vi "Format UI Size.vi"() -> (0 "error out":errorcluster)   [LabVIEW 2015, in "Configuration Tool.lvlib"]
uses:
  Configuration Tool.lvlib
  <vilib>/Utility/miscctls.llb/LVPositionTypeDef.ctl
  <vilib>/Utility/traverseref.llb/TRef TravTarget.ctl
  <vilib>/Utility/miscctls.llb/LVBoundsTypeDef.ctl
  <vilib>/Utility/traverseref.llb/VI Scripting - Traverse.lvlib
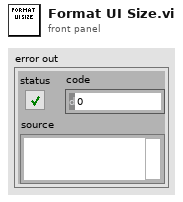
[diagram p1: front panel]
types:
  T1 = typedef "LVBoundsTypeDef.ctl" = cluster{"Width":u32, "Height":u32}
  T2 = typedef "TRef TravTarget.ctl" = enum16{"FP", "BD", "Other"}
  T3 = typedef "LVPositionTypeDef.ctl" = cluster{"Left":i32, "Top":i32}
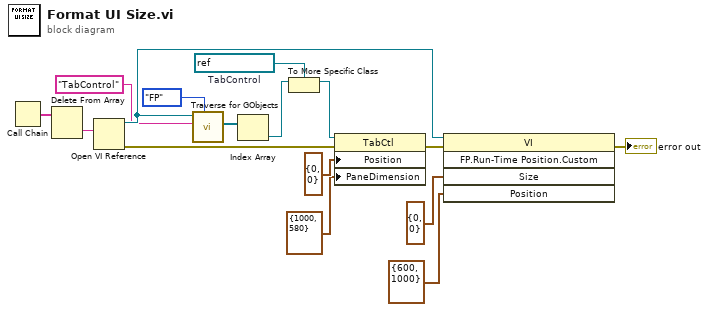
[diagram p0: block diagram]
diagram:
  w3 = refnum<vi> refnum  # TabControl
  n1 = Call Chain() -> (call chain=w11:string[])
  n2 = Delete From Array(array=w11) -> (deleted portion=w10:string)  [unwired: 2 in, 1 out]
  n3 = Open VI Reference(vi path=w10) -> (vi reference=w8:refnum<vi>, error out=w9:errorcluster)  [unwired: 5 in]
  n4 = call <vilib>:"Traverse for GObjects.vi"("Traverse Target"=TRef_TravTarget."FP", "Class Name"="TabControl", "VI Refnum"=w8) -> ("References"=w7:refnum<vi>[])  [unwired: 5 in, 3 out]
  n5 = Index Array(array=w7) -> (element=w4:refnum<vi>)  [unwired: 1 in]
  n6 = To More Specific Class(target class=w3, reference=w4) -> (specific class reference=w2:refnum<vi>)  [unwired: 1 in, 1 out]
  n7 = property on="Property Node" class="TabCtl"(reference=w2, error in=w9, "Position"=T3 {"Left"=0, "Top"=0}, "PaneDimension"=T1 {"Width"=1000, "Height"=580} ("Tab Control Pane Dimension")) -> (error out=w15:errorcluster)  [unwired: 1 out]
  n8 = invoke class="VI" method="FP.Run-Time Position.Custom"(reference=w8, error in=w15, "Size"=cluster{"Top":i16, "Left":i16} {"Top"=0, "Left"=0} ("Position"), "Position"=cluster{"Height":i16, "Width":i16} {"Height"=600, "Width"=1000} ("Size")) -> (error out=→"error out":errorcluster)  [unwired: 1 in, 4 out]
